vi "lfieldpanel_store_single_frame.vi"(7 "image_data":T1, 8 "error in (no error)":errorcluster, 9 "notes":string, 10 "Path":path, 11 "lightfield_panel in":refnum<class "lightfield_panel.lvclass">) -> (0 "error out":errorcluster, 3 "lightfield_panel out":refnum<class "lightfield_panel.lvclass">)   [LabVIEW 2015, in "lightfield_panel.lvclass"]
uses:
  lightfield_panel.lvclass
  lightfield_hdf5_logger_class/lfield_logger.lvclass
  lightfield_hdf5_logger_class/metadata_tdef.ctl
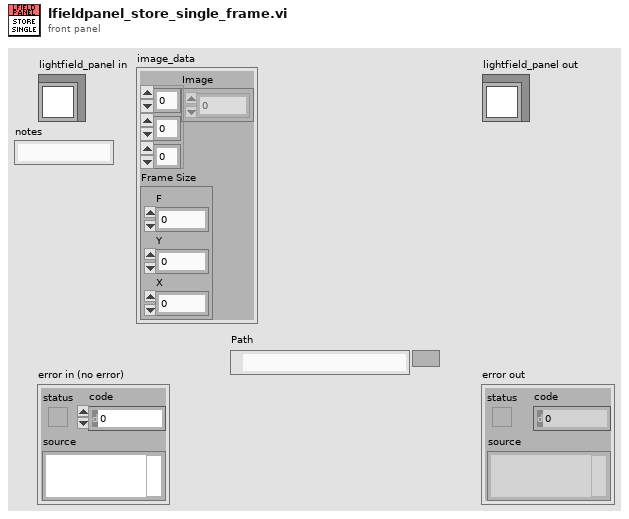
[diagram p1: front panel]
types:
  T1 = cluster{"Image":dbl[][][], "Frame Size":cluster{"F":i32, "Y":i32, "X":i32}}
  T2 = typedef "metadata_tdef.ctl" = cluster{"notes":string}
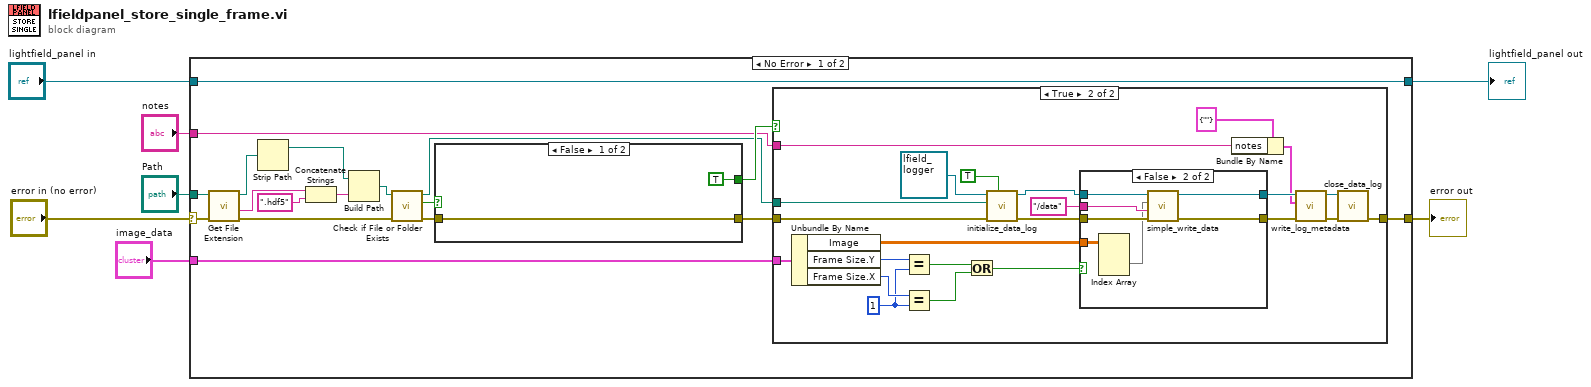
[diagram p0: block diagram]
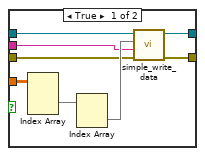
[diagram p3: hidden frame]
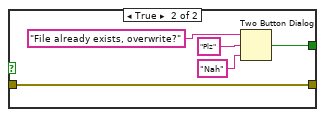
[diagram p4: hidden frame]
diagram:
  n1 = case shown="No Error" "error in (no error)" {
    selector: "error in (no error)" -> [w22 w73]
    tunnel: [w9 w73] -> w6
    tunnel: [w25 w72] -> w4
    tunnel: "lightfield_panel in" -> [w25 w72]
    tunnel: "image_data" -> [w24 _]
    tunnel: "Path" -> [w23 _]
    tunnel: "notes" -> [w8 _]
    frame No Error {
      n2 = call <vilib>:"Get File Extension.vi"("error in (no error)"=w22, "file"=w23) -> ("error out"=w15:errorcluster, "filename without extension"=w21:string, "dup file"=w19:path)  [unwired: 5 in, 2 out]
      n3 = Strip Path(path=w19) -> (stripped path=w18:path)  [unwired: 1 out]
      n4 = Concatenate Strings(w21, ".hdf5" ("string")) -> (w17:string)
      n5 = Build Path(base path=w18, name or relative path=w17) -> (appended path=w16:path)
      n6 = call <vilib>:"Check if File or Folder Exists.vi"("error in (no error)"=w15, "path"=w16) -> ("error out"=w12:errorcluster, "file or folder exists?"=w14:bool, "dup path"=w10:path)  [unwired: 7 in]
      n7 = case shown="False" w14 {
        tunnel: [TRUE ("T button?") w68] -> w13
        tunnel: w12 -> [w65 w67]
        tunnel: [w65 w67] -> w11
        frame False {
        }
        frame True {
          n8 = Two Button Dialog(message="File already exists, overwrite?", 1:"Nah" ("F button name (\"Cancel\")"), 2:"Plz" ("T button name (\"OK\")")) -> (T button?=w68:bool)
        }
      }
      n9 = case shown="True" w13 {
        tunnel: w24 -> [_ w49]
        tunnel: w11 -> [w26 w41]
        tunnel: w10 -> [_ w39]
        tunnel: [w26 w34] -> w9
        tunnel: w8 -> [_ w27]
        frame False {
        }
        frame True {
          w46 = 1 ("y")
          n10 = Unbundle By Name(w49) -> ("Image"=w42:dbl[][][], "Frame Size.Y"=w48:i32, "Frame Size.X"=w47:i32)
          n11 = Equal?(x=w48, y=w46) -> (x = y?=w44:bool)
          n12 = Equal?(x=w47, y=w46) -> (x = y?=w45:bool)
          n13 = Or(x=w44, y=w45) -> (x .or. y?=w43:bool)
          n14 = call-dynamic "initialize_data_log.vi"("Overwrite?"=TRUE, "error in (no error)"=w41, "Path"=w39, "lfield_logger in"=refnum<class "lfield_logger.lvclass"> refnum) -> ("error out"=w36:errorcluster, "lfield_logger out"=w37:refnum<class "lfield_logger.lvclass">)  [unwired: 6 in]
          n15 = case shown="False" w43 {
            tunnel: w42 -> [w57 w64]
            tunnel: w37 -> [w54 w63]
            tunnel: w36 -> [w53 w62]
            tunnel: "/data" -> [w52 w61]
            tunnel: [w51 w60] -> w30
            tunnel: [w50 w59] -> w33
            frame True {
              n16 = Index Array(array=w57) -> (element=w56:dbl[][])  [unwired: 3 in]
              n17 = Index Array(array=w56) -> (element=w55:dbl[])  [unwired: 2 in]
              n18 = call "simple_write_data.vi"("error in (no error)"=w53, "path"=w52, "Data"=w55, "lfield_logger in"=w54) -> ("error out"=w50:errorcluster, "lfield_logger out"=w51:refnum<class "lfield_logger.lvclass">)  [unwired: 6 in]
            }
            frame False {
              n19 = Index Array(array=w64) -> (element=w58:dbl[][])  [unwired: 3 in]
              n20 = call "simple_write_data.vi"("error in (no error)"=w62, "path"=w61, "Data"=w58, "lfield_logger in"=w63) -> ("error out"=w59:errorcluster, "lfield_logger out"=w60:refnum<class "lfield_logger.lvclass">)  [unwired: 6 in]
            }
          }
          n21 = Bundle By Name(cluster=T2 {"notes"=""} ("output cluster"), "notes"=w27) -> (w28:T2)
          n22 = call-dynamic "write_log_metadata.vi"("error in (no error)"=w33, "data"=w28, "lfield_logger in"=w30) -> ("error out"=w32:errorcluster, "lfield_logger out"=w31:refnum<class "lfield_logger.lvclass">)  [unwired: 7 in]
          n23 = call-dynamic "close_data_log.vi"("error in (no error)"=w32, "lfield_logger in"=w31) -> ("error out"=w34:errorcluster)  [unwired: 8 in, 1 out]
        }
      }
    }
    frame Error {
    }
  }
  "error out" <- w6
  "lightfield_panel out" <- w4
